vi "Configure Master Scan Interval Group.vi"(0 "VISA resource name":refnum<visa-resource-name>, 9 "Scan Group No.(1)":i32=1 min=1 max=2, 11 "error in (no error)":errorcluster) -> (4 "VISA resource name out":refnum<visa-resource-name>, 15 "error out":errorcluster)   [LabVIEW 2020, in "Yokogawa GX Series.lvlib"]
doc: "Sets scan master interval group.\n\nCommand: SMasterScanGrp.\n\nNote: This command is valid when recorder is in dual interval mode."
uses:
  <instrlib>/Yokogawa GX Series/Yokogawa GX Series.lvlib
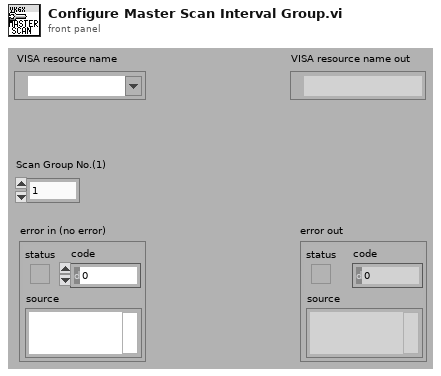
[diagram p1: front panel]
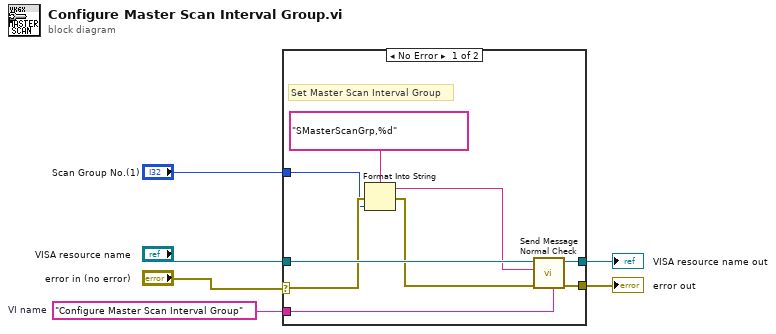
[diagram p0: block diagram]
diagram:
  w2 = "Configure Master Scan Interval Group"  # VI name
  n1 = case shown="No Error" "error in (no error)" {
    selector: "error in (no error)" -> [w10 w16]
    tunnel: [w15 w17] -> w6
    tunnel: [w14 w16] -> w5
    tunnel: "VISA resource name" -> [w13 w17]
    tunnel: w2 -> [w9 _]
    tunnel: "Scan Group No.(1)" -> [w7 _]
    frame No Error {
      # "Set Master Scan Interval Group"
      n2 = Format Into String(format string="SMasterScanGrp,%d", error in=w10, w7) -> (resulting string=w8:string, error out=w11:errorcluster)  [unwired: 1 in]
      n3 = call <instrlib>:"Send Message Normal Check.vi"("Source (\"\")"=w9, "error in (no error)"=w11, "Send Message (\"\")"=w8, "VISA resource name"=w13) -> ("error out"=w14:errorcluster, "VISA resource name out"=w15:refnum<visa-resource-name>)  [unwired: 2 in, 4 out]
    }
    frame Error {
    }
  }
  "error out" <- w5
  "VISA resource name out" <- w6
